vi "Ring handler.vi"(8 "error in (no error)":errorcluster, 11 "Message Queues out":T1) -> (0 "error out":errorcluster, 3 "Message Queue":refnum<queue>)   [LabVIEW 2014]
uses:
  support/Message Queue/All Message Queues.ctl
  support/Message Queue/Message Cluster.ctl
  Time Out.ctl
  Digital/Digital Input Cluster.ctl
  Digital/Enum DO.ctl
  Engine/Message.ctl
  Teszt/Teszt.ctl
  Teszt/Command.ctl
  <vilib>/Utility/miscctls.llb/LVRectTypeDef.ctl
  support/Message Queue/Enqueue Message (Single).vi
  <vilib>/Utility/error.llb/Error Cluster From Error Code.vi
  <vilib>/ErrorRing/Error Ring.xnode
  support/Message Queue/Message Queue.lvlib
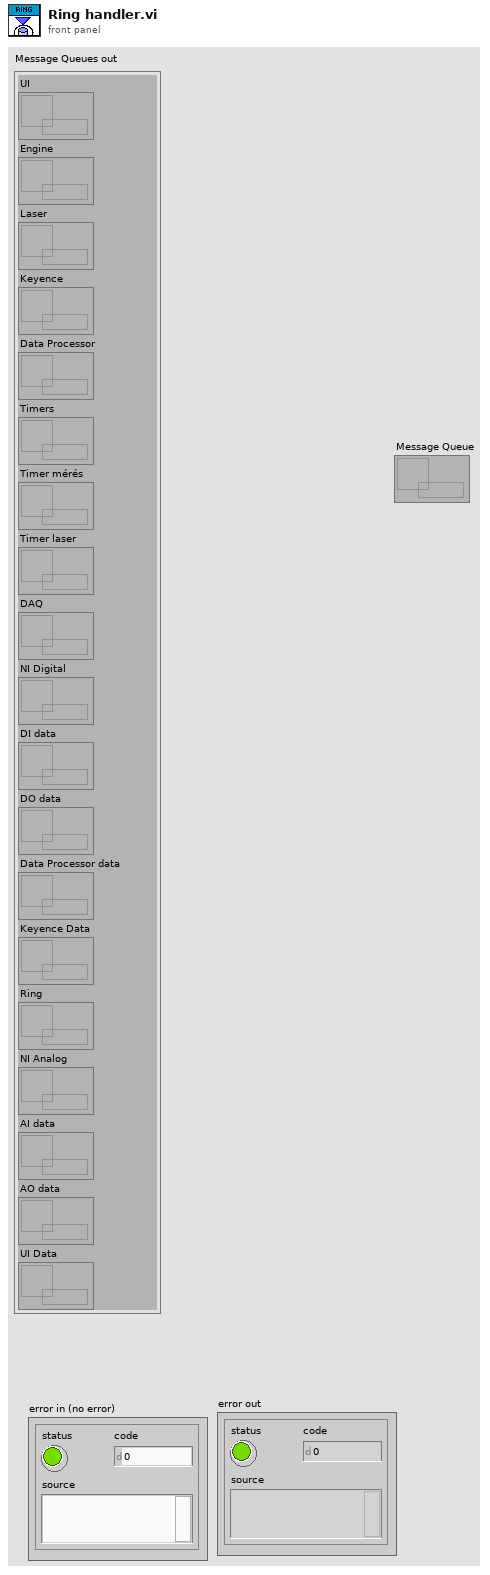
[diagram p1: front panel]
types:
  T1 = typedef "Message Queue.lvlib/All Message Queues.ctl" = cluster{"UI":refnum<queue>, "Engine":refnum<queue>, "Laser":refnum<queue>, "Keyence":refnum<queue>, "Data Processor":refnum<queue>, "Timers":refnum<queue>, "Timer mérés":refnum<queue>, "Timer laser":refnum<queue>, "DAQ":refnum<queue>, "NI Digital":refnum<queue>, "DI data":refnum<queue>, "DO data":refnum<queue>, "Data Processor data":refnum<queue>, "Keyence Data":refnum<queue>, "Ring":refnum<queue>, "NI Analog":refnum<queue>, "AI data":refnum<queue>, "AO data":refnum<queue>, "UI Data":refnum<queue>}
  T2 = typedef "Time Out.ctl" = cluster{"Time Out Reset":bool, "Timed Out":bool, "Time Out Time (s)":dbl}
  T3 = typedef "Enum DO.ctl" = enum16{"Izolációs relé", "B oldal relé (nincs használva)", "48V relé", "Elszívás KI", "Bördelezés teszt", "Gyûrû megnyomás", "Termék rögzítés", "R mérés relé", "200mA relé", "NTC mérés relé", "Levegõ BE"}
  T4 = typedef "LVRectTypeDef.ctl" = cluster{"Left":i16, "Top":i16, "Right":i16, "Bottom":i16}
  T5 = typedef "Digital Input Cluster.ctl" = cluster{"PCIE-6321 IN":cluster{"Termék bördelezve":bool, "Izolációs relék OK":bool, "Rézgyûrû a terméken":bool, "Termék rögzítve":bool, "Termék a gyûrûzõben":bool, "Rézgyûrû behelyezve":bool, "Rézgyûrû elengedve":bool, "Rézgyûrû megnyomva":bool, "Termék elengedve":bool, "Levegõ rendben":bool, "Termék jelen (táv)":bool, "Termék jelen (fém)":bool, "Selejt érzékelõ":bool}}
  T6 = typedef "Teszt.ctl" = cluster{"Thread ID":dbl, "Mérésszám":string, "Mérés/Utasítás":string, "Command":T7, "Min":string, "Max":string, "Aktív?":bool, "Log?":bool, "Kiértékelés":bool, "Etalon 1 exp":bool, "Etalon 2 exp":bool, "Etalon 3 exp":bool, "Etalon 4 exp":bool, "Etalon 5 exp":bool}
  T7 = typedef "Command.ctl" = cluster{"Parancs":string, "Paraméter 1":string, "Paraméter 2":string, "Paraméter 3":string, "Paraméter 4":string, "Paraméter 5":string, "Eredmény":string}
  T8 = typedef "Message.ctl" = cluster{"Thread ID":u16, "Callback":string, "Data":variant, "Error":errorcluster}
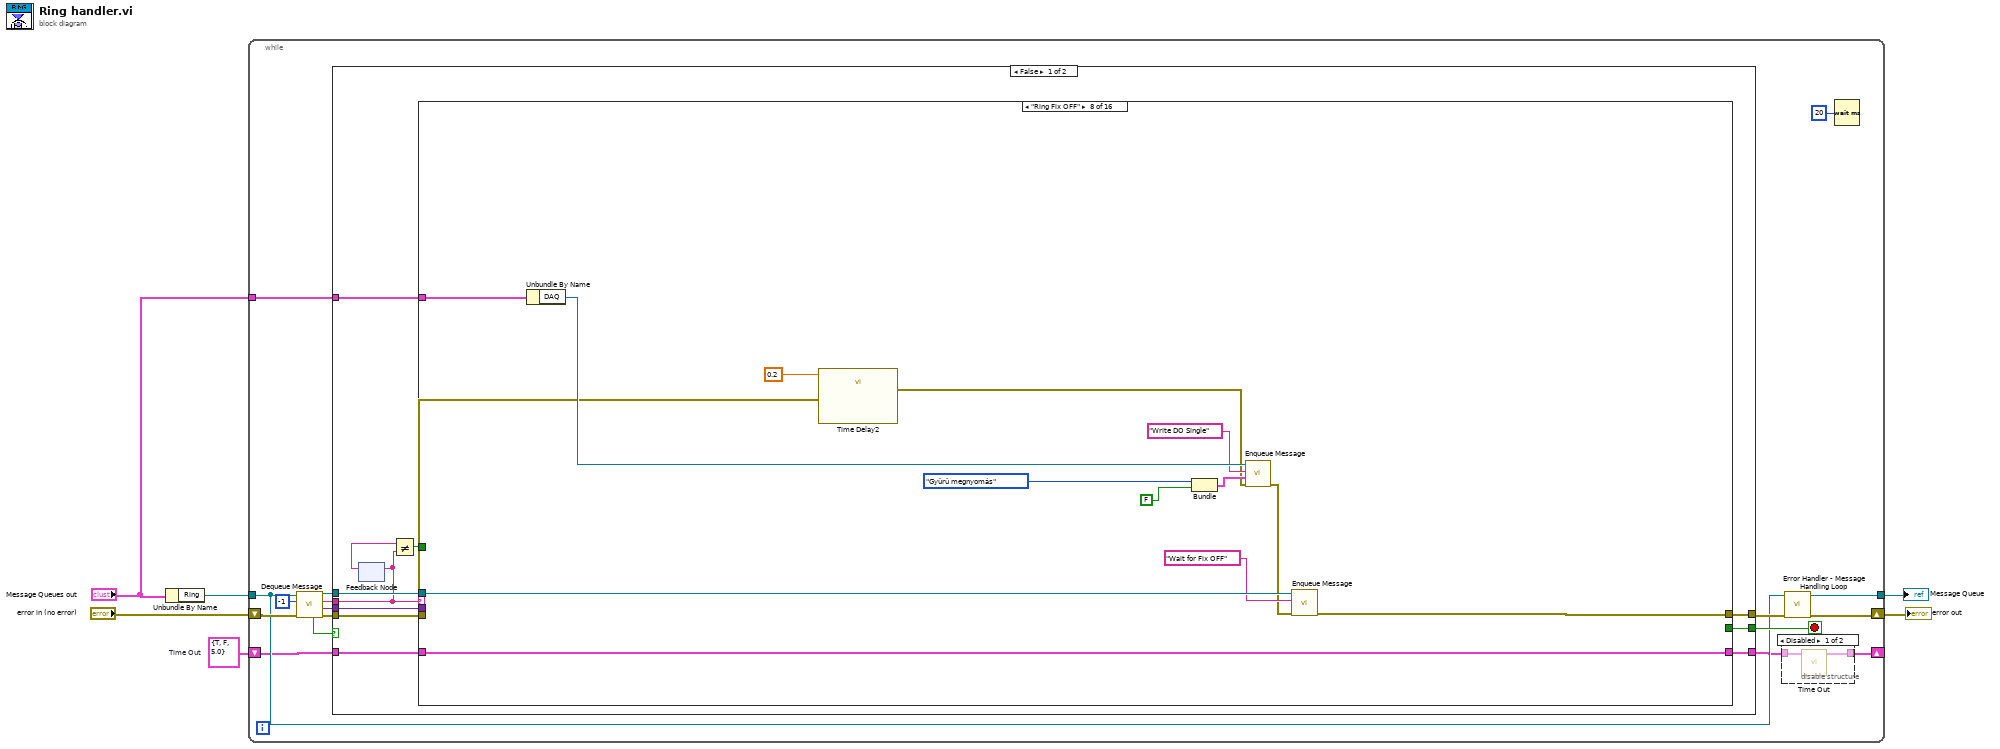
[diagram p0: block diagram]
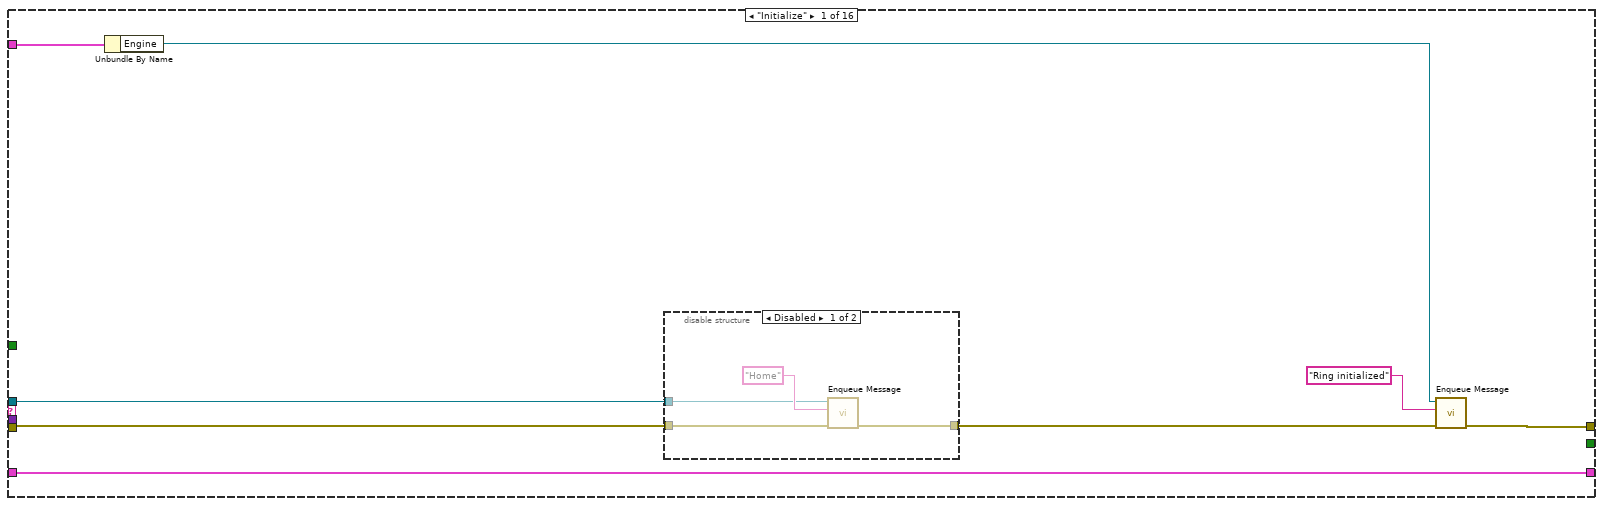
[diagram p3: hidden frame]
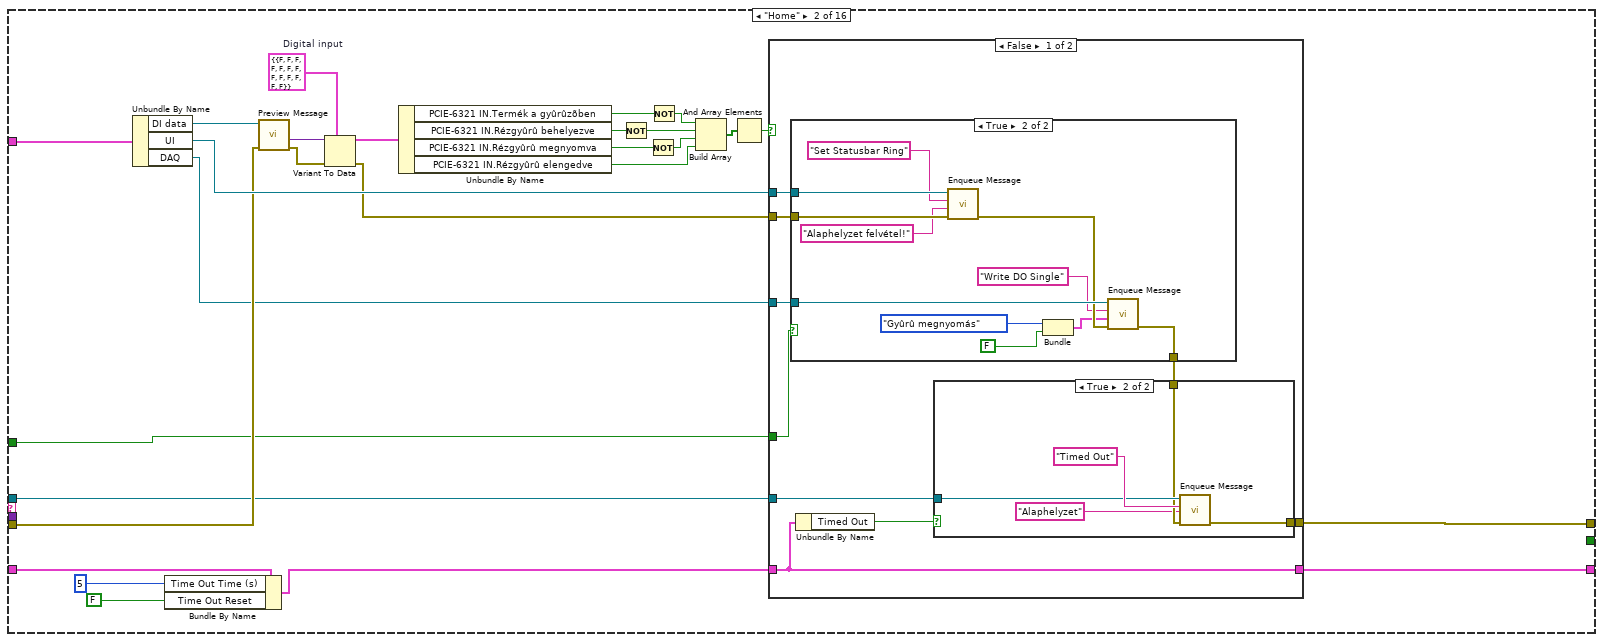
[diagram p5: hidden frame]
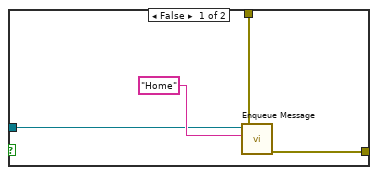
[diagram p7: hidden frame]
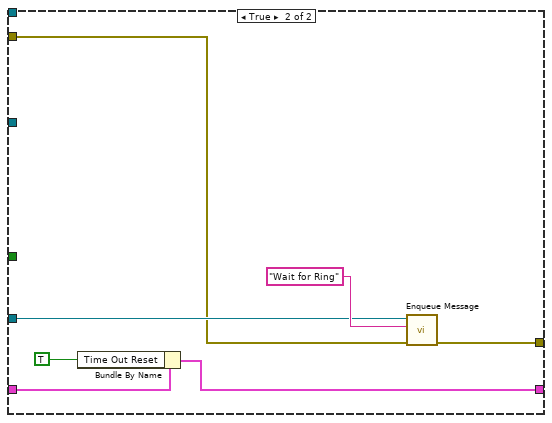
[diagram p8: hidden frame]
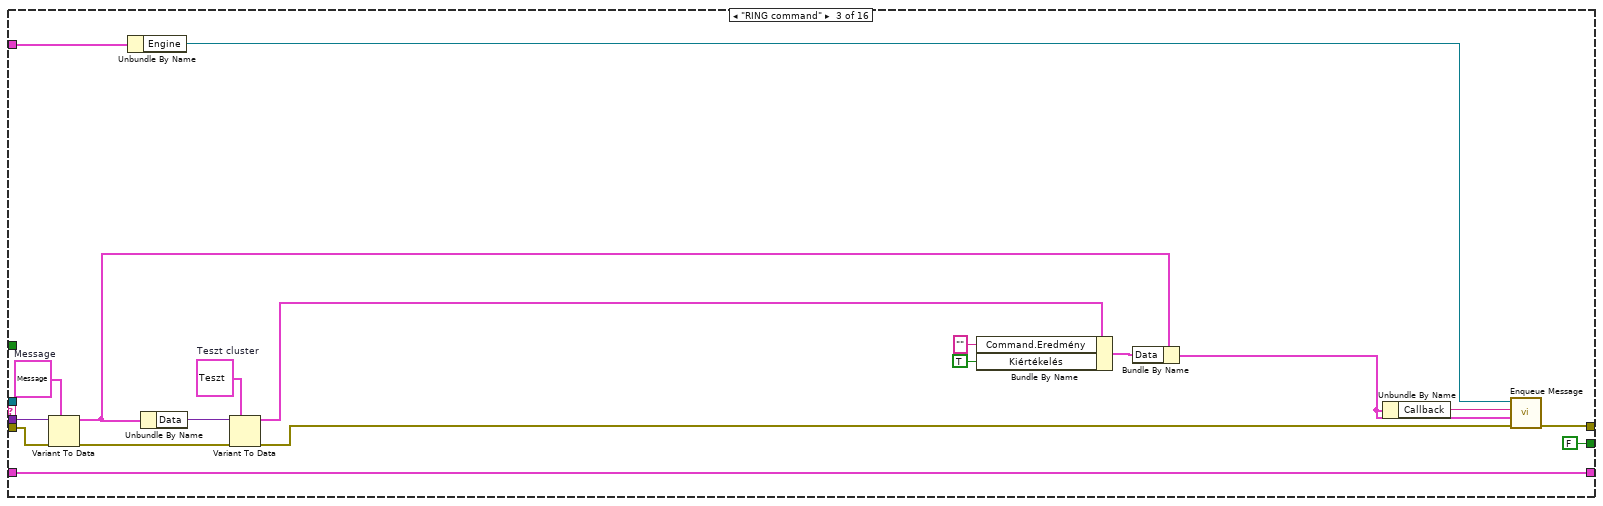
[diagram p9: hidden frame]
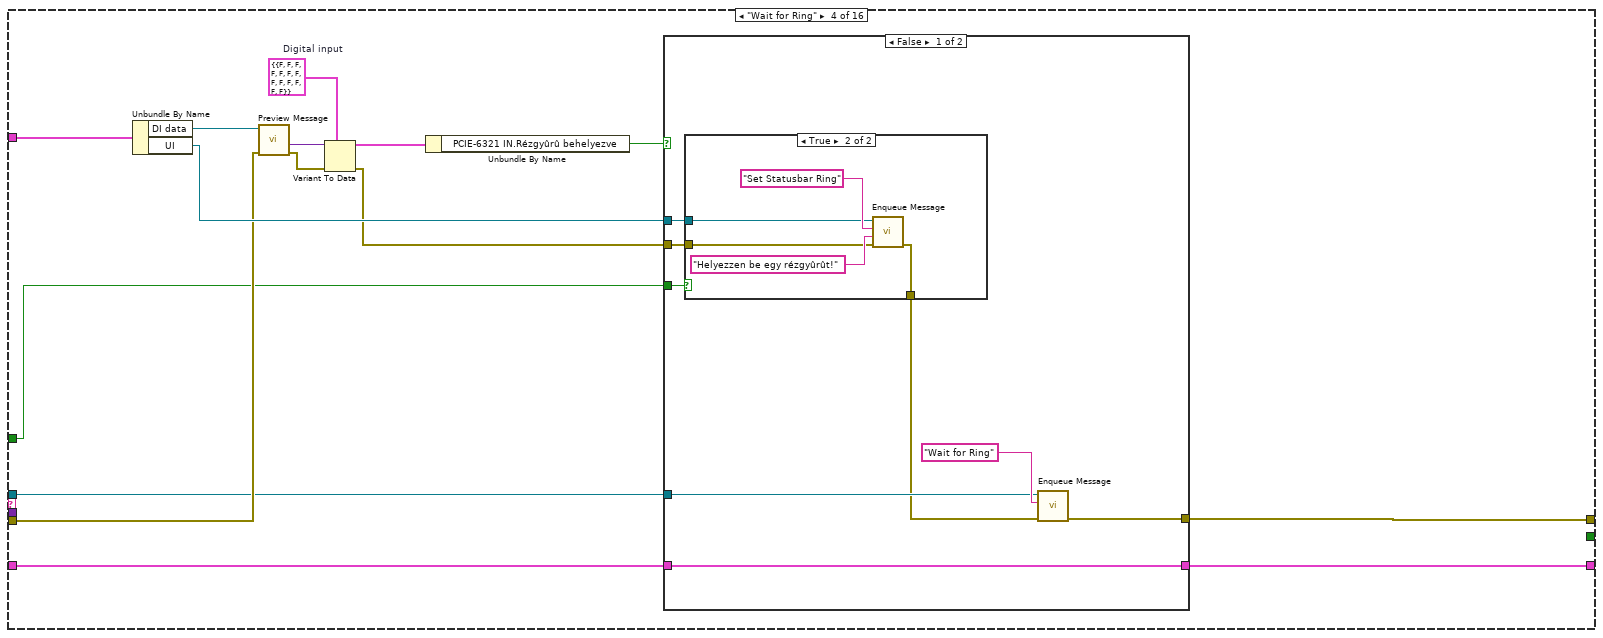
[diagram p10: hidden frame]
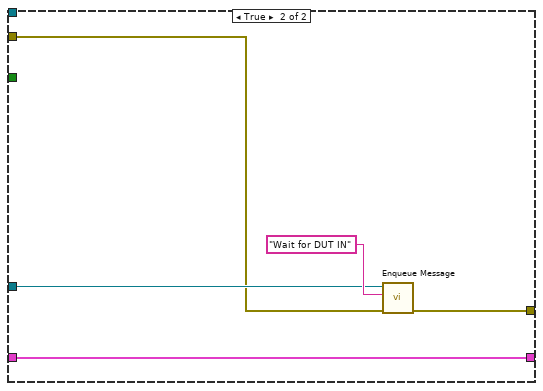
[diagram p12: hidden frame]
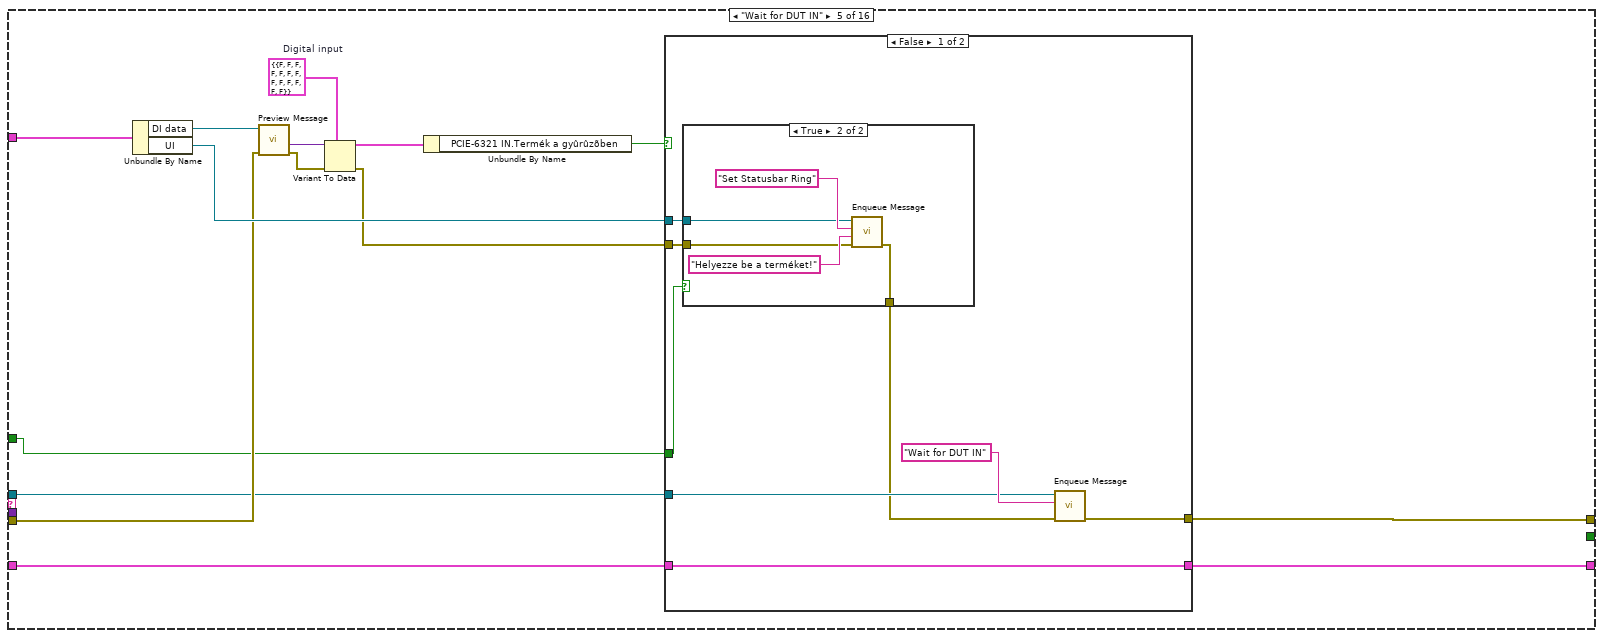
[diagram p13: hidden frame]
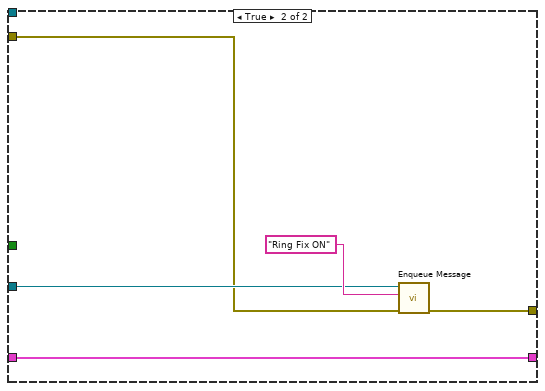
[diagram p15: hidden frame]
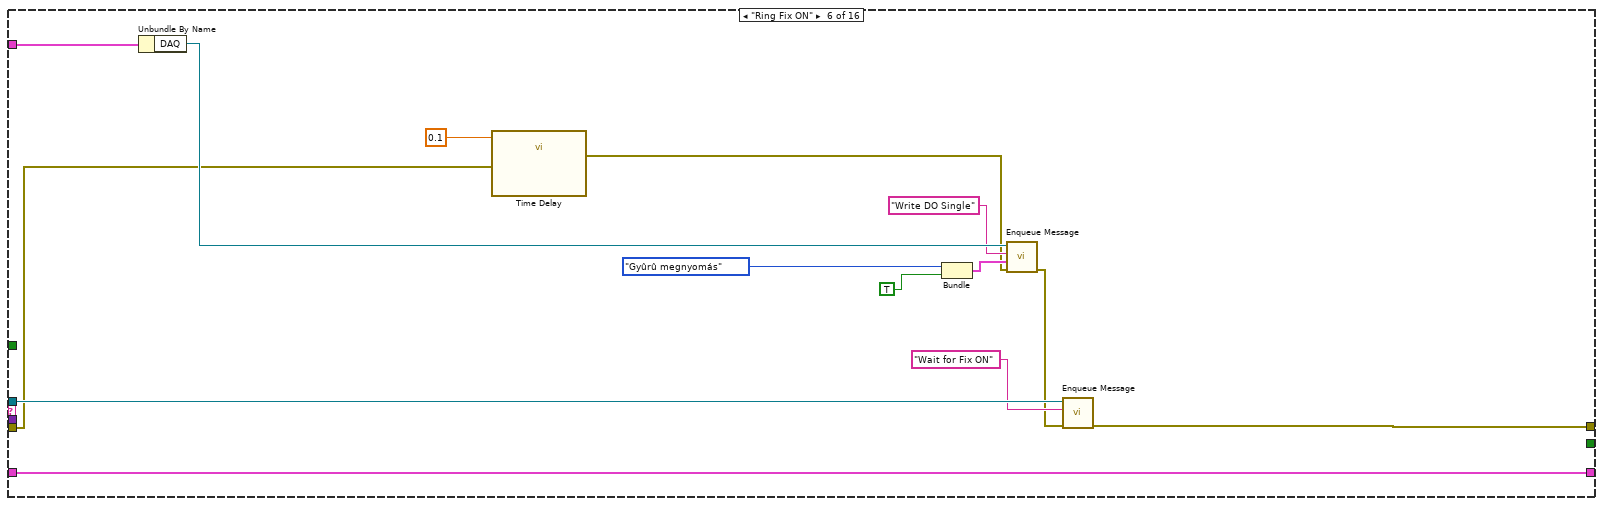
[diagram p16: hidden frame]
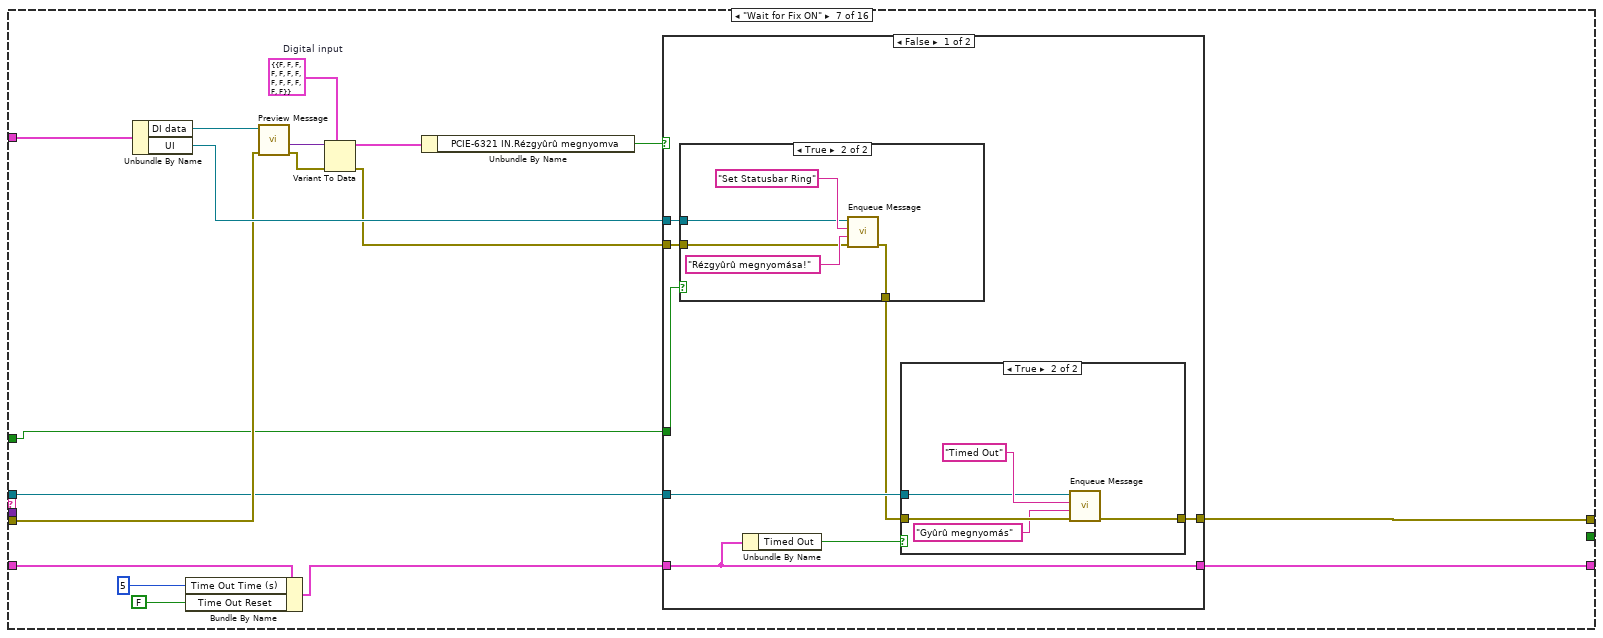
[diagram p17: hidden frame]
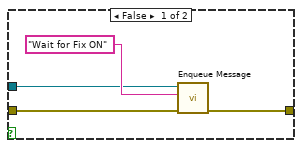
[diagram p19: hidden frame]
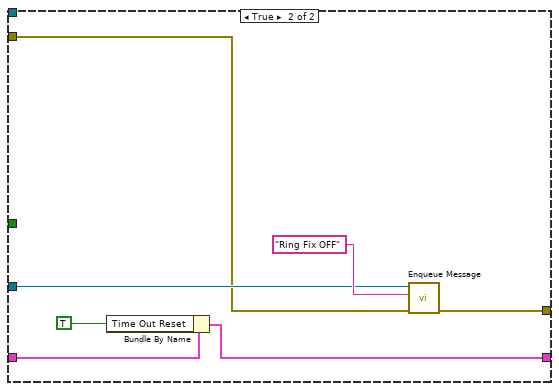
[diagram p20: hidden frame]
diagram:
  w1 = T2 {"Time Out Reset"=TRUE, "Timed Out"=FALSE, "Time Out Time (s)"=5.0}  # Time Out
  n1 = Unbundle By Name("Message Queues out") -> ("Ring"=w3:refnum<queue>)
  n2 = while {
    tunnel: w3 -> [w11]
    shift-right: [w15] -> w6
    shift-left: "error in (no error)" -> [w23]
    tunnel: "Message Queues out" -> [w13]
    tunnel: [w12] -> w2
    shift-right: [w10] -> _
    shift-left: w1 -> [w9]
    stop <- w19 stop-if-true
    n3 = call "Dequeue Message.vi"("error in (no error)"=w23, "timeout in ms (-1)"=-1, "Message Queue"=w11) -> ("error out"=w21:errorcluster, "Message Data"=w16:variant, "Message"=w22:string, "dup Message Queue"=w20:refnum<queue>, "timed out?"=w17:bool)  [unwired: 4 in]
    n4 = case shown="False" w17 {
      tunnel: w22 -> [w29 _]
      tunnel: w21 -> [w37 w440]
      tunnel: w20 -> [w36 _]
      tunnel: [w35 FALSE] -> w19
      tunnel: [w34 w440] -> w14
      tunnel: w16 -> [w33 _]
      tunnel: w13 -> [w32 _]
      tunnel: w9 -> [w31 w439]
      tunnel: [w30 w439] -> w8
      frame False {
        n5 = feedback #1() -> (w28:string)  [unwired: 1 in]
        n6 = feedback-in #1(w29) -> ()
        n7 = Not Equal?(x=w28, y=w29) -> (x != y?=w27:bool)
        n8 = case shown="\"Ring Fix OFF\"" w29 {
          selector: w29 -> [_ _ _ _ _ _ _ _ _ _ _ _ _ _ _ w429]
          tunnel: w37 -> [w41 w71 w125 w141 w175 w206 w226 w268 w288 w333 w375 w388 w406 w421 w425 _]
          tunnel: w36 -> [w39 w57 _ w137 w171 w212 w223 w274 w284 w329 w374 w380 w409 w420 w427 _]
          tunnel: [w44 w68 w132 w138 w172 w214 w224 w276 w285 w330 w373 w378 w410 w422 w424 w430] -> w34
          tunnel: [_ _ FALSE _ _ _ _ _ _ _ _ _ _ _ TRUE FALSE] -> w35
          tunnel: w33 -> [_ _ w124 _ _ _ _ _ _ _ _ w387 w407 _ _ _]
          tunnel: w32 -> [w43 w77 w130 w148 w182 w215 w233 w277 w295 w340 _ w395 w408 _ _ _]
          tunnel: w31 -> [w38 w56 w115 w136 w170 w203 w220 w265 w282 w328 w372 w393 w405 w417 w423 w428]
          tunnel: [w38 w53 w115 w135 w169 w203 w221 w265 w283 w327 w372 w392 w405 w417 w423 w428] -> w30
          tunnel: w27 -> [_ w51 _ w134 w168 _ w216 _ w278 w326 _ _ _ _ _ _]
          frame "Initialize" {
            n9 = Unbundle By Name(w43) -> ("Engine"=w42:refnum<queue>)
            n10 = disable-structure shown="Disabled" {
              disable-tunnel: w41 -> [w48 w50]
              disable-tunnel: [w47 w50] -> w40
              disable-tunnel: w39 -> [w46 _]
              frame Disabled {
                n11 = call-poly "Enqueue Message.vi"("error in (no error)"=w48, "Message"="Home", "Message Queue"=w46) -> ("error out"=w47:errorcluster)  [unwired: 7 in, 1 out]
              }
              frame Enabled {
              }
            }
            n12 = call-poly "Enqueue Message.vi"("error in (no error)"=w40, "Message"="Ring initialized", "Message Queue"=w42) -> ("error out"=w44:errorcluster)  [unwired: 7 in, 1 out]
          }
          frame "Home" {
            w76 = T5 {"PCIE-6321 IN"={"Termék bördelezve"=FALSE, "Izolációs relék OK"=FALSE, "Rézgyûrû a terméken"=FALSE, "Termék rögzítve"=FALSE, "Termék a gyûrûzõben"=FALSE, "Rézgyûrû behelyezve"=FALSE, "Rézgyûrû elengedve"=FALSE, "Rézgyûrû megnyomva"=FALSE, "Termék elengedve"=FALSE, "Levegõ rendben"=FALSE, "Termék jelen (táv)"=FALSE, "Termék jelen (fém)"=FALSE, "Selejt érzékelõ"=FALSE}}  # Digital input
            n13 = Unbundle By Name(w77) -> ("DI data"=w75:refnum<queue>, "UI"=w72:refnum<queue>, "DAQ"=w67:refnum<queue>)
            n14 = Bundle By Name(cluster=w56, "Time Out Time (s)"=5 ("Reset"), "Time Out Reset"=FALSE ("Reset")) -> (w52:T2)
            n15 = call "Preview Message.vi"("error in (no error)"=w71, "Message Queue"=w75) -> ("error out"=w70:errorcluster, "Message Data"=w74:variant)  [unwired: 5 in, 3 out]
            n16 = Variant To Data(error in=w70, type=w76, Variant=w74) -> (data=w73:T5, error out=w69:errorcluster)
            n17 = Unbundle By Name(w73) -> ("PCIE-6321 IN.Termék a gyûrûzõben"=w61:bool, "PCIE-6321 IN.Rézgyûrû behelyezve"=w62:bool, "PCIE-6321 IN.Rézgyûrû megnyomva"=w63:bool, "PCIE-6321 IN.Rézgyûrû elengedve"=w58:bool)
            n18 = Not(x=w62) -> (.not. x?=w60:bool)
            n19 = Not(x=w63) -> (.not. x?=w66:bool)
            n20 = Not(x=w61) -> (.not. x?=w59:bool)
            n21 = Build Array(w59, w60, w66, w58) -> (w64:bool[])
            n22 = And Array Elements(Boolean array=w64) -> (logical AND=w65:bool)
            n23 = case shown="False" w65 {
              tunnel: w72 -> [w86 _]
              tunnel: w69 -> [w85 w111]
              tunnel: [w84 w113] -> w68
              tunnel: w67 -> [w83 _]
              tunnel: w57 -> [w81 w112]
              tunnel: [w79 w109] -> w53
              tunnel: w52 -> [w79 w110]
              tunnel: w51 -> [w78 _]
              frame False {
                n24 = case shown="True" w78 {
                  tunnel: w86 -> [_ w98]
                  tunnel: w85 -> [w87 w97]
                  tunnel: w83 -> [_ w96]
                  tunnel: [w87 w94] -> w82
                  frame False {
                  }
                  frame True {
                    n25 = call-poly "Enqueue Message.vi"("error in (no error)"=w97, "Message Data"="Alaphelyzet felvétel!" ("Message"), "Message"="Set Statusbar Ring", "Message Queue"=w98) -> ("error out"=w95:errorcluster)  [unwired: 6 in, 1 out]
                    n26 = Bundle("Enum"=Enum_DO."Gyûrû megnyomás", FALSE) -> (w92:cluster{"Enum":T3, bool})  [unwired: 1 in]
                    n27 = call-poly "Enqueue Message.vi"("error in (no error)"=w95, "Message Data"=w92, "Message"="Write DO Single", "Message Queue"=w96) -> ("error out"=w94:errorcluster)  [unwired: 6 in, 1 out]
                  }
                }
                n28 = Unbundle By Name(w79) -> ("Timed Out"=w80:bool)
                n29 = case shown="True" w80 {
                  tunnel: [w101 w104] -> w84
                  tunnel: w82 -> [w100 w105]
                  tunnel: w81 -> [w99 w106]
                  frame False {
                    n30 = call-poly "Enqueue Message.vi"("error in (no error)"=w100, "Message"="Home", "Message Queue"=w99) -> ("error out"=w101:errorcluster)  [unwired: 7 in, 1 out]
                  }
                  frame True {
                    n31 = call-poly "Enqueue Message.vi"("error in (no error)"=w105, "Message Data"="Alaphelyzet" ("Message"), "Message"="Timed Out", "Message Queue"=w106) -> ("error out"=w104:errorcluster)  [unwired: 6 in, 1 out]
                  }
                }
              }
              frame True {
                n32 = Bundle By Name(cluster=w110, "Time Out Reset"=TRUE ("Reset")) -> (w109:T2)
                n33 = call-poly "Enqueue Message.vi"("error in (no error)"=w111, "Message"="Wait for Ring", "Message Queue"=w112) -> ("error out"=w113:errorcluster)  [unwired: 7 in, 1 out]
              }
            }
          }
          frame "RING command" {
            w126 = T6 {"Thread ID"=0.0, "Mérésszám"="", "Mérés/Utasítás"="", "Command"={"Parancs"="", "Paraméter 1"="", "Paraméter 2"="", "Paraméter 3"="", "Paraméter 4"="", "Paraméter 5"="", "Eredmény"=""}, "Min"="", "Max"="", "Aktív?"=FALSE, "Log?"=FALSE, "Kiértékelés"=FALSE, "Etalon 1 exp"=FALSE, "Etalon 2 exp"=FALSE, "Etalon 3 exp"=FALSE, "Etalon 4 exp"=FALSE, "Etalon 5 exp"=FALSE}  # Teszt cluster
            w129 = T8 {"Thread ID"=0, "Callback"="", "Data"=variant, "Error"={"status"=FALSE, "code"=0, "source"=""}}  # Message
            n34 = Variant To Data(error in=w125, type=w129, Variant=w124) -> (data=w120:T8, error out=w128:errorcluster)
            n35 = Unbundle By Name(w130) -> ("Engine"=w131:refnum<queue>)
            n36 = Unbundle By Name(w120) -> ("Data"=w127:variant)
            n37 = Variant To Data(error in=w128, type=w126, Variant=w127) -> (data=w116:T6, error out=w119:errorcluster)
            n38 = Bundle By Name(cluster=w116, "Command.Eredmény"="", "Kiértékelés"=TRUE) -> (w123:T6)
            n39 = Bundle By Name(cluster=w120, "Data"=w123) -> (w121:T8)
            n40 = Unbundle By Name(w121) -> ("Callback"=w122:string)
            n41 = call-poly "Enqueue Message.vi"("error in (no error)"=w119, "Message Data"=w121, "Message"=w122, "Message Queue"=w131) -> ("error out"=w132:errorcluster)  [unwired: 6 in, 1 out]
          }
          frame "Wait for Ring" {
            w147 = T5 {"PCIE-6321 IN"={"Termék bördelezve"=FALSE, "Izolációs relék OK"=FALSE, "Rézgyûrû a terméken"=FALSE, "Termék rögzítve"=FALSE, "Termék a gyûrûzõben"=FALSE, "Rézgyûrû behelyezve"=FALSE, "Rézgyûrû elengedve"=FALSE, "Rézgyûrû megnyomva"=FALSE, "Termék elengedve"=FALSE, "Levegõ rendben"=FALSE, "Termék jelen (táv)"=FALSE, "Termék jelen (fém)"=FALSE, "Selejt érzékelõ"=FALSE}}  # Digital input
            n42 = Unbundle By Name(w148) -> ("DI data"=w146:refnum<queue>, "UI"=w142:refnum<queue>)
            n43 = call "Preview Message.vi"("error in (no error)"=w141, "Message Queue"=w146) -> ("error out"=w140:errorcluster, "Message Data"=w145:variant)  [unwired: 5 in, 3 out]
            n44 = Variant To Data(error in=w140, type=w147, Variant=w145) -> (data=w144:T5, error out=w139:errorcluster)
            n45 = Unbundle By Name(w144) -> ("PCIE-6321 IN.Rézgyûrû behelyezve"=w143:bool)
            n46 = case shown="False" w143 {
              tunnel: w137 -> [w154 w166]
              tunnel: w142 -> [w156 _]
              tunnel: w139 -> [w153 w164]
              tunnel: [w151 w165] -> w138
              tunnel: w136 -> [w150 w163]
              tunnel: [w150 w163] -> w135
              tunnel: w134 -> [w149 _]
              frame False {
                n47 = case shown="True" w149 {
                  tunnel: w156 -> [_ w160]
                  tunnel: w153 -> [w157 w159]
                  tunnel: [w157 w158] -> w152
                  frame False {
                  }
                  frame True {
                    n48 = call-poly "Enqueue Message.vi"("error in (no error)"=w159, "Message Data"="Helyezzen be egy rézgyûrût!" ("Message"), "Message"="Set Statusbar Ring", "Message Queue"=w160) -> ("error out"=w158:errorcluster)  [unwired: 6 in, 1 out]
                  }
                }
                n49 = call-poly "Enqueue Message.vi"("error in (no error)"=w152, "Message"="Wait for Ring", "Message Queue"=w154) -> ("error out"=w151:errorcluster)  [unwired: 7 in, 1 out]
              }
              frame True {
                n50 = call-poly "Enqueue Message.vi"("error in (no error)"=w164, "Message"="Wait for DUT IN", "Message Queue"=w166) -> ("error out"=w165:errorcluster)  [unwired: 7 in, 1 out]
              }
            }
          }
          frame "Wait for DUT IN" {
            w181 = T5 {"PCIE-6321 IN"={"Termék bördelezve"=FALSE, "Izolációs relék OK"=FALSE, "Rézgyûrû a terméken"=FALSE, "Termék rögzítve"=FALSE, "Termék a gyûrûzõben"=FALSE, "Rézgyûrû behelyezve"=FALSE, "Rézgyûrû elengedve"=FALSE, "Rézgyûrû megnyomva"=FALSE, "Termék elengedve"=FALSE, "Levegõ rendben"=FALSE, "Termék jelen (táv)"=FALSE, "Termék jelen (fém)"=FALSE, "Selejt érzékelõ"=FALSE}}  # Digital input
            n51 = Unbundle By Name(w182) -> ("DI data"=w180:refnum<queue>, "UI"=w176:refnum<queue>)
            n52 = call "Preview Message.vi"("error in (no error)"=w175, "Message Queue"=w180) -> ("error out"=w174:errorcluster, "Message Data"=w179:variant)  [unwired: 5 in, 3 out]
            n53 = Variant To Data(error in=w174, type=w181, Variant=w179) -> (data=w178:T5, error out=w173:errorcluster)
            n54 = Unbundle By Name(w178) -> ("PCIE-6321 IN.Termék a gyûrûzõben"=w177:bool)
            n55 = case shown="False" w177 {
              tunnel: w171 -> [w188 w200]
              tunnel: w176 -> [w190 _]
              tunnel: w173 -> [w187 w198]
              tunnel: [w185 w199] -> w172
              tunnel: w170 -> [w184 w197]
              tunnel: [w184 w197] -> w169
              tunnel: w168 -> [w183 _]
              frame False {
                n56 = case shown="True" w183 {
                  tunnel: w190 -> [_ w194]
                  tunnel: w187 -> [w191 w193]
                  tunnel: [w191 w192] -> w186
                  frame False {
                  }
                  frame True {
                    n57 = call-poly "Enqueue Message.vi"("error in (no error)"=w193, "Message Data"="Helyezze be a terméket!" ("Message"), "Message"="Set Statusbar Ring", "Message Queue"=w194) -> ("error out"=w192:errorcluster)  [unwired: 6 in, 1 out]
                  }
                }
                n58 = call-poly "Enqueue Message.vi"("error in (no error)"=w186, "Message"="Wait for DUT IN", "Message Queue"=w188) -> ("error out"=w185:errorcluster)  [unwired: 7 in, 1 out]
              }
              frame True {
                n59 = call-poly "Enqueue Message.vi"("error in (no error)"=w198, "Message"="Ring Fix ON", "Message Queue"=w200) -> ("error out"=w199:errorcluster)  [unwired: 7 in, 1 out]
              }
            }
          }
          frame "Ring Fix ON" {
            n60 = Unbundle By Name(w215) -> ("DAQ"=w213:refnum<queue>)
            n61 = call "Time Delay"("error in (no error)"=w206, "Delay Time (s)"=0.1) -> ("error out"=w204:errorcluster)  [unwired: 9 in]
            n62 = Bundle("Enum"=Enum_DO."Gyûrû megnyomás", TRUE) -> (w209:cluster{"Enum":T3, bool})  [unwired: 1 in]
            n63 = call-poly "Enqueue Message.vi"("error in (no error)"=w204, "Message Data"=w209, "Message"="Write DO Single", "Message Queue"=w213) -> ("error out"=w207:errorcluster)  [unwired: 6 in, 1 out]
            n64 = call-poly "Enqueue Message.vi"("error in (no error)"=w207, "Message"="Wait for Fix ON", "Message Queue"=w212) -> ("error out"=w214:errorcluster)  [unwired: 7 in, 1 out]
          }
          frame "Wait for Fix ON" {
            w232 = T5 {"PCIE-6321 IN"={"Termék bördelezve"=FALSE, "Izolációs relék OK"=FALSE, "Rézgyûrû a terméken"=FALSE, "Termék rögzítve"=FALSE, "Termék a gyûrûzõben"=FALSE, "Rézgyûrû behelyezve"=FALSE, "Rézgyûrû elengedve"=FALSE, "Rézgyûrû megnyomva"=FALSE, "Termék elengedve"=FALSE, "Levegõ rendben"=FALSE, "Termék jelen (táv)"=FALSE, "Termék jelen (fém)"=FALSE, "Selejt érzékelõ"=FALSE}}  # Digital input
            n65 = Unbundle By Name(w233) -> ("DI data"=w231:refnum<queue>, "UI"=w227:refnum<queue>)
            n66 = Bundle By Name(cluster=w220, "Time Out Time (s)"=5 ("Reset"), "Time Out Reset"=FALSE ("Reset")) -> (w219:T2)
            n67 = call "Preview Message.vi"("error in (no error)"=w226, "Message Queue"=w231) -> ("error out"=w225:errorcluster, "Message Data"=w230:variant)  [unwired: 5 in, 3 out]
            n68 = Variant To Data(error in=w225, type=w232, Variant=w230) -> (data=w229:T5, error out=w222:errorcluster)
            n69 = Unbundle By Name(w229) -> ("PCIE-6321 IN.Rézgyûrû megnyomva"=w228:bool)
            n70 = case shown="False" w228 {
              tunnel: w223 -> [w240 w262]
              tunnel: w227 -> [w241 _]
              tunnel: w222 -> [w239 w260]
              tunnel: [w237 w261] -> w224
              tunnel: w219 -> [w236 w258]
              tunnel: [w236 w257] -> w221
              tunnel: w216 -> [w234 _]
              frame False {
                n71 = case shown="True" w234 {
                  tunnel: w241 -> [_ w245]
                  tunnel: w239 -> [w242 w244]
                  tunnel: [w242 w243] -> w238
                  frame False {
                  }
                  frame True {
                    n72 = call-poly "Enqueue Message.vi"("error in (no error)"=w244, "Message Data"="Rézgyûrû megnyomása!" ("Message"), "Message"="Set Statusbar Ring", "Message Queue"=w245) -> ("error out"=w243:errorcluster)  [unwired: 6 in, 1 out]
                  }
                }
                n73 = Unbundle By Name(w236) -> ("Timed Out"=w235:bool)
                n74 = case shown="True" w235 {
                  tunnel: w240 -> [w250 w255]
                  tunnel: w238 -> [w249 w254]
                  tunnel: [w248 w253] -> w237
                  frame False {
                    n75 = call-poly "Enqueue Message.vi"("error in (no error)"=w249, "Message"="Wait for Fix ON", "Message Queue"=w250) -> ("error out"=w248:errorcluster)  [unwired: 7 in, 1 out]
                  }
                  frame True {
                    n76 = call-poly "Enqueue Message.vi"("error in (no error)"=w254, "Message Data"="Gyûrû megnyomás" ("Message"), "Message"="Timed Out", "Message Queue"=w255) -> ("error out"=w253:errorcluster)  [unwired: 6 in, 1 out]
                  }
                }
              }
              frame True {
                n77 = Bundle By Name(cluster=w258, "Time Out Reset"=TRUE ("Reset")) -> (w257:T2)
                n78 = call-poly "Enqueue Message.vi"("error in (no error)"=w260, "Message"="Ring Fix OFF", "Message Queue"=w262) -> ("error out"=w261:errorcluster)  [unwired: 7 in, 1 out]
              }
            }
          }
          frame "Ring Fix OFF" {
            n79 = Unbundle By Name(w277) -> ("DAQ"=w275:refnum<queue>)
            n80 = call "Time Delay2"("error in (no error)"=w268, "Delay Time (s)"=0.2) -> ("error out"=w266:errorcluster)  [unwired: 9 in]
            n81 = Bundle("Enum"=Enum_DO."Gyûrû megnyomás", FALSE) -> (w271:cluster{"Enum":T3, bool})  [unwired: 1 in]
            n82 = call-poly "Enqueue Message.vi"("error in (no error)"=w266, "Message Data"=w271, "Message"="Write DO Single", "Message Queue"=w275) -> ("error out"=w269:errorcluster)  [unwired: 6 in, 1 out]
            n83 = call-poly "Enqueue Message.vi"("error in (no error)"=w269, "Message"="Wait for Fix OFF", "Message Queue"=w274) -> ("error out"=w276:errorcluster)  [unwired: 7 in, 1 out]
          }
          frame "Wait for Fix OFF" {
            w294 = T5 {"PCIE-6321 IN"={"Termék bördelezve"=FALSE, "Izolációs relék OK"=FALSE, "Rézgyûrû a terméken"=FALSE, "Termék rögzítve"=FALSE, "Termék a gyûrûzõben"=FALSE, "Rézgyûrû behelyezve"=FALSE, "Rézgyûrû elengedve"=FALSE, "Rézgyûrû megnyomva"=FALSE, "Termék elengedve"=FALSE, "Levegõ rendben"=FALSE, "Termék jelen (táv)"=FALSE, "Termék jelen (fém)"=FALSE, "Selejt érzékelõ"=FALSE}}  # Digital input
            n84 = Unbundle By Name(w295) -> ("DI data"=w293:refnum<queue>, "UI"=w289:refnum<queue>)
            n85 = Bundle By Name(cluster=w282, "Time Out Time (s)"=5 ("Reset"), "Time Out Reset"=FALSE ("Reset")) -> (w281:T2)
            n86 = call "Preview Message.vi"("error in (no error)"=w288, "Message Queue"=w293) -> ("error out"=w287:errorcluster, "Message Data"=w292:variant)  [unwired: 5 in, 3 out]
            n87 = Variant To Data(error in=w287, type=w294, Variant=w292) -> (data=w291:T5, error out=w286:errorcluster)
            n88 = Unbundle By Name(w291) -> ("PCIE-6321 IN.Rézgyûrû elengedve"=w290:bool)
            n89 = case shown="False" w290 {
              tunnel: w284 -> [w302 w324]
              tunnel: w289 -> [w303 _]
              tunnel: w286 -> [w301 w322]
              tunnel: [w299 w323] -> w285
              tunnel: w281 -> [w297 w321]
              tunnel: [w297 w320] -> w283
              tunnel: w278 -> [w296 _]
              frame False {
                n90 = case shown="True" w296 {
                  tunnel: w303 -> [_ w307]
                  tunnel: w301 -> [w304 w306]
                  tunnel: [w304 w305] -> w300
                  frame False {
                  }
                  frame True {
                    n91 = call-poly "Enqueue Message.vi"("error in (no error)"=w306, "Message Data"="Rézgyûrû megnyomása!" ("Message"), "Message"="Set Statusbar Ring", "Message Queue"=w307) -> ("error out"=w305:errorcluster)  [unwired: 6 in, 1 out]
                  }
                }
                n92 = Unbundle By Name(w297) -> ("Timed Out"=w298:bool)
                n93 = case shown="True" w298 {
                  tunnel: w302 -> [w312 w315]
                  tunnel: w300 -> [w311 w316]
                  tunnel: [w310 w317] -> w299
                  frame False {
                    n94 = call-poly "Enqueue Message.vi"("error in (no error)"=w311, "Message"="Wait for Fix OFF", "Message Queue"=w312) -> ("error out"=w310:errorcluster)  [unwired: 7 in, 1 out]
                  }
                  frame True {
                    n95 = call-poly "Enqueue Message.vi"("error in (no error)"=w316, "Message Data"="Gyûrû elengedés" ("Message"), "Message"="Timed Out", "Message Queue"=w315) -> ("error out"=w317:errorcluster)  [unwired: 6 in, 1 out]
                  }
                }
              }
              frame True {
                n96 = Bundle By Name(cluster=w321, "Time Out Reset"=TRUE) -> (w320:T2)
                n97 = call-poly "Enqueue Message.vi"("error in (no error)"=w322, "Message"="Wait for DUT OUT", "Message Queue"=w324) -> ("error out"=w323:errorcluster)  [unwired: 7 in, 1 out]
              }
            }
          }
          frame "Wait for DUT OUT" {
            w339 = T5 {"PCIE-6321 IN"={"Termék bördelezve"=FALSE, "Izolációs relék OK"=FALSE, "Rézgyûrû a terméken"=FALSE, "Termék rögzítve"=FALSE, "Termék a gyûrûzõben"=FALSE, "Rézgyûrû behelyezve"=FALSE, "Rézgyûrû elengedve"=FALSE, "Rézgyûrû megnyomva"=FALSE, "Termék elengedve"=FALSE, "Levegõ rendben"=FALSE, "Termék jelen (táv)"=FALSE, "Termék jelen (fém)"=FALSE, "Selejt érzékelõ"=FALSE}}  # Digital input
            n98 = Unbundle By Name(w340) -> ("DI data"=w338:refnum<queue>, "UI"=w334:refnum<queue>)
            n99 = call "Preview Message.vi"("error in (no error)"=w333, "Message Queue"=w338) -> ("error out"=w332:errorcluster, "Message Data"=w337:variant)  [unwired: 5 in, 3 out]
            n100 = Variant To Data(error in=w332, type=w339, Variant=w337) -> (data=w336:T5, error out=w331:errorcluster)
            n101 = Unbundle By Name(w336) -> ("PCIE-6321 IN.Termék a gyûrûzõben"=w335:bool)
            n102 = case shown="True" w335 {
              tunnel: w329 -> [w356 w363]
              tunnel: w334 -> [w350 w365]
              tunnel: w331 -> [w353 w362]
              tunnel: [w352 w360] -> w330
              tunnel: w328 -> [w341 w359]
              tunnel: [w341 w359] -> w327
              tunnel: w326 -> [_ w358]
              frame False {
                w347 = T8 {"Thread ID"=0, "Callback"="", "Data"=variant, "Error"={"status"=FALSE, "code"=0, "source"=""}}  # Message
                n103 = call-poly "Enqueue Message.vi"("error in (no error)"=w353, "Message Data"="" ("Message"), "Message"="Set Statusbar Ring", "Message Queue"=w350) -> ("error out"=w349:errorcluster)  [unwired: 6 in, 1 out]
                n104 = Bundle By Name(cluster=w347, "Data"=TRUE, "Thread ID"=u16 1) -> (w346:T8)
                n105 = call-poly "Enqueue Message.vi"("error in (no error)"=w349, "Message Data"=w346, "Message"="Kiértékelés Ring UI", "Message Queue"=w350) -> ("error out"=w343:errorcluster)  [unwired: 6 in, 1 out]
                n106 = call "Time Delay3"("error in (no error)"=w343, "Delay Time (s)"=1.0) -> ("error out"=w342:errorcluster)  [unwired: 9 in]
                n107 = call-poly "Enqueue Message.vi"("error in (no error)"=w342, "Message"="Home", "Message Queue"=w356) -> ("error out"=w352:errorcluster)  [unwired: 7 in, 1 out]
              }
              frame True {
                n108 = case shown="True" w358 {
                  tunnel: w365 -> [_ w369]
                  tunnel: w362 -> [w366 w368]
                  tunnel: [w366 w367] -> w361
                  frame False {
                  }
                  frame True {
                    n109 = call-poly "Enqueue Message.vi"("error in (no error)"=w368, "Message Data"="Vegye ki a terméket!" ("Message"), "Message"="Set Statusbar Ring", "Message Queue"=w369) -> ("error out"=w367:errorcluster)  [unwired: 6 in, 1 out]
                  }
                }
                n110 = call-poly "Enqueue Message.vi"("error in (no error)"=w361, "Message"="Wait for DUT OUT", "Message Queue"=w363) -> ("error out"=w360:errorcluster)  [unwired: 7 in, 1 out]
              }
            }
          }
          frame "Abort" {
            n111 = Flush Queue(queue=w374, error in (no error)=w375) -> (error out=w373:errorcluster)  [unwired: 2 out]
          }
          frame "Timed Out" {
            # "Ablak méret\n385\n250"
            n112 = Variant To Data(type="" ("Message"), Variant=w387) -> (data=w376:string)  [unwired: 1 in, 1 out]
            n113 = Unbundle By Name(w395) -> ("UI"=w390:refnum<queue>)
            n114 = call <vilib>:"Space Constant.vi"() -> ("String"=w384:string)
            n115 = Concatenate Strings("Timed Out" ("Message"), w384, w376) -> (w381:string)
            n116 = call-poly "Enqueue Message.vi"("error in (no error)"=w388, "Message Data"=w381, "Message"="Set Statusbar Ring", "Message Queue"=w390) -> ("error out"=w389:errorcluster)  [unwired: 6 in, 1 out]
            n117 = case shown="Default" w376 {
              tunnel: w390 -> [_ w399]
              tunnel: w389 -> [w396 w398]
              tunnel: [w396 w397] -> w383
              frame "Alaphelyzet" {
              }
              frame Default {
                w402 = T8 {"Thread ID"=0, "Callback"="", "Data"=variant, "Error"={"status"=FALSE, "code"=0, "source"=""}}  # Message
                n118 = Bundle By Name(cluster=w402, "Data"=FALSE, "Thread ID"=u16 1) -> (w401:T8)
                n119 = call-poly "Enqueue Message.vi"("error in (no error)"=w398, "Message Data"=w401, "Message"="Kiértékelés Ring UI", "Message Queue"=w399) -> ("error out"=w397:errorcluster)  [unwired: 6 in, 1 out]
              }
            }
            n120 = Bundle By Name(cluster=w393, "Time Out Reset"=TRUE ("Reset")) -> (w392:T2)
            n121 = call "Dialog Window Time Out.vi"("Front Panel Window:Panel Bounds"=T4 {"Left"=260, "Top"=260, "Right"=645, "Bottom"=510}, "Üzenet be"=w381, "Error In"=w383) -> ("Error Out"=w379:errorcluster)  [unwired: 8 in]
            n122 = call-poly "Enqueue Message.vi"("error in (no error)"=w379, "Message"="Home", "Message Queue"=w380) -> ("error out"=w378:errorcluster)  [unwired: 7 in, 1 out]
          }
          frame "Error" {
            n123 = Unbundle By Name(w408) -> ("UI"=w413:refnum<queue>)
            n124 = call-poly "Enqueue Message.vi"("error in (no error)"=w406, "Message Data"=w407, "Message"="Error", "Message Queue"=w413) -> ("error out"=w415:errorcluster)  [unwired: 6 in, 1 out]
            n125 = call-poly "Enqueue Message.vi"("Priority Message? (F)"=TRUE, "error in (no error)"=w406, "Message"="Initiate Stop", "Message Queue"=w409) -> ("error out"=w414:errorcluster)  [unwired: 6 in, 1 out]
            n126 = Merge Errors(w415, w414) -> (w410:errorcluster)
          }
          frame "Initiate Stop" {
            n127 = call-poly "Enqueue Message.vi"("Priority Message? (F)"=TRUE, "error in (no error)"=w421, "Message"="Program Stop", "Message Queue"=w420) -> ("error out"=w422:errorcluster)  [unwired: 6 in, 1 out]
          }
          frame "Program Stop" {
            n128 = Flush Queue(queue=w427, error in (no error)=w425) -> (error out=w424:errorcluster)  [unwired: 2 out]
          }
          frame Default {
            n129 = xnode "Error Ring"("parameter 0"=w429) -> ("error out"=w430:errorcluster)
          }
        }
      }
      frame True {
      }
    }
    n130 = disable-structure shown="Disabled" {
      disable-tunnel: [w25 w26] -> w10
      disable-tunnel: w8 -> [w24 w26]
      frame Disabled {
        n131 = call "Time Out.vi"("Time Out in"=w24) -> ("Time Out out"=w25:T2)  [unwired: 10 in]
      }
      frame Enabled {
      }
    }
    n132 = call "Error Handler - Message Handling Loop.vi"("error in (no error)"=w14, "Message Queue"=w11) -> ("dup error in"=w15:errorcluster, "dup Message Queue"=w12:refnum<queue>)  [unwired: 8 in]
    n133 = Wait (ms)(milliseconds to wait=u32 20) -> ()  [unwired: 1 out]
  }
  "error out" <- w6
  "Message Queue" <- w2
